vi "CANOpen_Scan Device List.vi"(10 "Baud Rate":T1 items=["1 Mbit/s"=0, "800 kbit/s"=1, "500 kbit/s"=2, "250 kbit/s"=3, "125 kbit/s"=4, "50 kbit/s"=6, "20 kbit/s"=7, "10 kbit/s"=8], 11 "CANOpen Interface Name":T2 items=["CANopen01", "CANopen02", "CANopen03", "CANopen04", "CANopen05", "CANopen06", "CANopen07", "CANopen08", "CANopen09", "CANopen10", "CANopen11", "CANopen12", "CANopen13", "CANopen14", "CANopen15", "CANopen16", "CANopen17", "CANopen18", "CANopen19", "CANopen20", "CANopen21", "CANopen22", "CANopen23", "CANopen24", "CANopen25", "CANopen26", "CANopen27", "CANopen28", "CANopen29", "CANopen30", "CANopen31", "CANopen32"]) -> ()   [LabVIEW 2013, in "CANOpen Addon Custom Device.lvlib"]
uses:
  CANOpen Addon Custom Device.lvlib
  Shared Code/CANOpen Interface Name.ctl
  <vilib>/CANopenLib/CANOPEN.llb/CANopen BaudRate.ctl
  <vilib>/CANopenLib/CANOPEN.llb/CANopen Interface Close.vi
  <vilib>/CANopenLib/CANOPEN.llb/CANopen Interface Create.vi
  <vilib>/CANopenLib/CANOPEN.llb/CANopen SDO Create.vi
  <vilib>/CANopenLib/CANOPEN.llb/CANopen SDO Read [U32].vi
  <vilib>/CANopenLib/CANOPEN.llb/CANopen SDO Close.vi
  <vilib>/CANopenLib/CANOPEN.llb/CANopen SDO Read [STR].vi
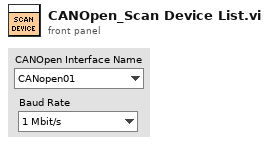
[diagram p1: front panel]
types:
  T1 = typedef "CANopen BaudRate.ctl" = u32
  T2 = typedef "CANOpen Addon Custom Device.lvlib/CANOpen Interface Name.ctl" = u32
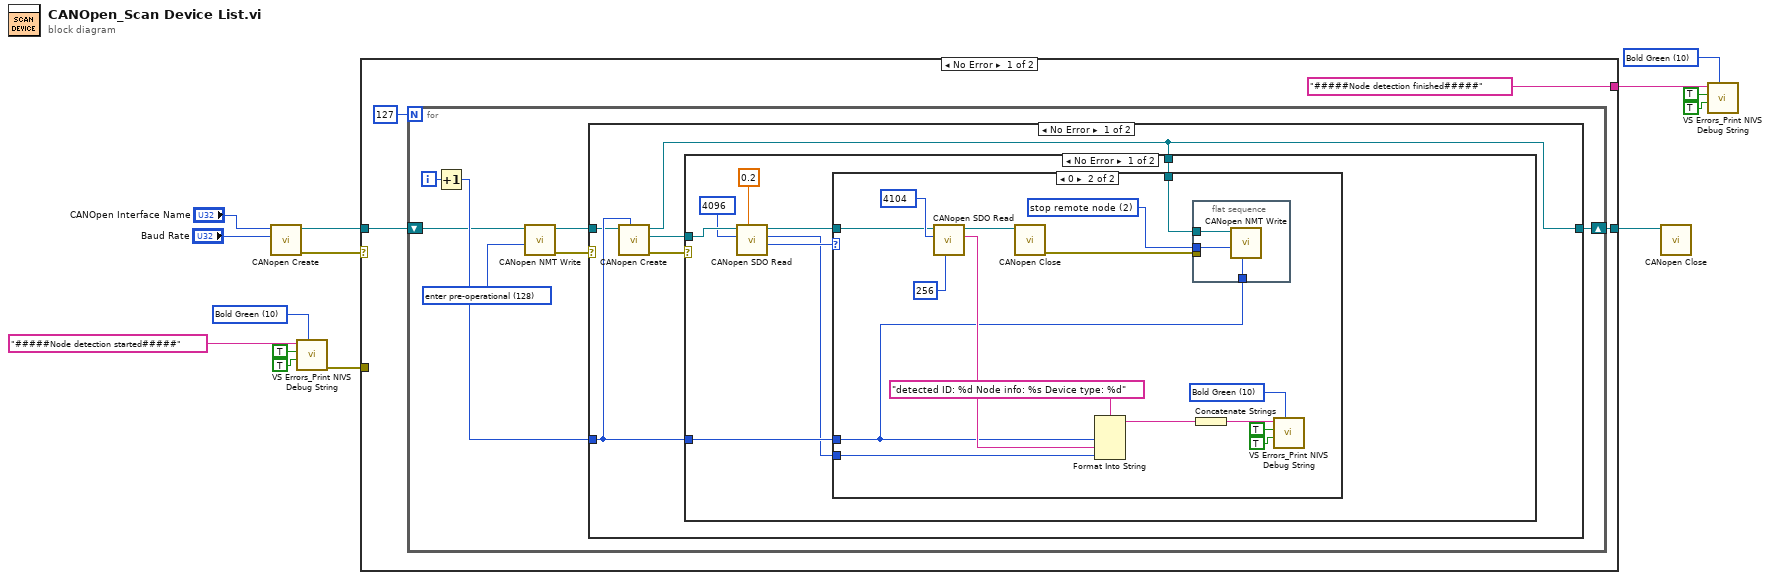
[diagram p0: block diagram]
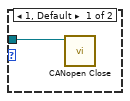
[diagram p2: hidden frame]
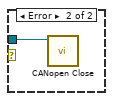
[diagram p3: hidden frame]
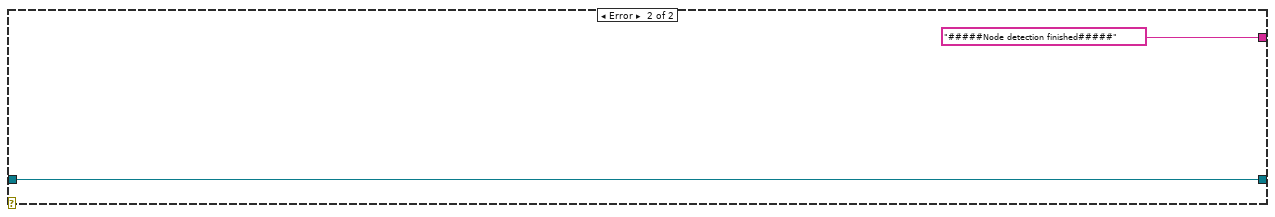
[diagram p5: hidden frame]
diagram:
  w4 = u16 10 items=["Plain White"=7, "Bold White"=15, "Bold Blue"=9, "Bold Green"=10, "Bold Red"=12] ("Color (Plain White)")
  w6 = u16 10 items=["Plain White"=7, "Bold White"=15, "Bold Blue"=9, "Bold Green"=10, "Bold Red"=12] ("Color (Plain White)")
  n1 = call-poly <vilib>:"CANopen Create.vi"("baud rate"="Baud Rate", "interface name"="CANOpen Interface Name") -> ("error out"=w10:errorcluster, "interface object out"=w12:refnum<k20>)  [unwired: 8 in]
  n2 = call "VS Errors_Print NIVS Debug String.vi"("Color (Plain White)"=w6, "Add to NIVS Log FIle? (T)"=TRUE, "Append EOL? (T)"=TRUE, "Debug String"="#####Node detection started#####") -> ("error out"=w7:errorcluster)  [unwired: 6 in]
  n3 = case shown="No Error" w10 {
    tunnel: w12 -> [w18 w62]
    tunnel: [w16 w62] -> w11
    tunnel: w7 -> [_ _]
    tunnel: ["#####Node detection finished#####" ("Debug String") "#####Node detection finished#####" ("Debug String")] -> w1
    frame No Error {
      n4 = for {
        N: 127 -> [_]
        shift-right: [w19] -> w16
        shift-left: w18 -> [w21]
        i -> [w25]
        w23 = u16 128 items=["start remote node"=1, "stop remote node"=2, "enter pre-operational"=128, "reset node"=129, "reset communication"=130] ("command")
        n5 = Increment(x=w25) -> (x+1=w24:i32)
        n6 = call <vilib>:"CANopen NMT Write.vi"("command"=w23, "interface object in"=w21) -> ("error out"=w20:errorcluster, "interface object out"=w22:refnum<k20>)  [unwired: 8 in]
        n7 = case shown="No Error" w20 {
          tunnel: w24 -> [w30 _]
          tunnel: w22 -> [w29 w60]
          tunnel: [w26 w60] -> w19
          frame No Error {
            n8 = call-poly <vilib>:"CANopen Create.vi"("node-ID"=w30, "interface object in"=w29) -> ("error out"=w27:errorcluster, "SDO object out"=w28:refnum<k20>, "interface object out"=w26:refnum<k20>)  [unwired: 7 in]
            n9 = case shown="No Error" w27 {
              tunnel: w30 -> [w38 _]
              tunnel: w28 -> [w37 w59]
              tunnel: w26 -> [w33 _]
              frame No Error {
                n10 = call-poly <vilib>:"CANopen SDO Read.vi"("timeout (1s)"=0.2, "object index"=u16 4096 ("Object Index"), "SDO object in"=w37) -> ("completion code"=w32:u32, "U32 data"=w31:u32, "SDO object out"=w34:refnum<k20>)  [unwired: 5 in, 1 out]
                n11 = case shown="0" w32 {
                  tunnel: w38 -> [_ w41]
                  tunnel: w34 -> [w39 w46]
                  tunnel: w33 -> [_ w43]
                  tunnel: w31 -> [_ w40]
                  frame 1, Default {
                    n12 = call-poly <vilib>:"CANopen Close.vi"("SDO object in"=w39) -> ()  [unwired: 10 in, 1 out]
                  }
                  frame 0 {
                    w42 = u16 2 items=["start remote node"=1, "stop remote node"=2, "enter pre-operational"=128, "reset node"=129, "reset communication"=130] ("command")
                    w53 = u16 10 items=["Plain White"=7, "Bold White"=15, "Bold Blue"=9, "Bold Green"=10, "Bold Red"=12] ("Color (Plain White)")
                    n13 = call-poly <vilib>:"CANopen SDO Read.vi"("data size"=u32 256, "object index"=u16 4104 ("Object Index"), "SDO object in"=w46) -> ("string data"=w45:string, "SDO object out"=w47:refnum<k20>)  [unwired: 5 in, 2 out]
                    n14 = call-poly <vilib>:"CANopen Close.vi"("SDO object in"=w47) -> ("error out"=w44:errorcluster)  [unwired: 10 in]
                    n15 = Format Into String(format string="detected ID: %d Node info: %s Device type: %d", w41, w45, w40) -> (resulting string=w54:string)  [unwired: 2 in, 1 out]
                    n16 = flat-sequence {
                      tunnel: w44 -> [_]
                      tunnel: w43 -> [w58]
                      tunnel: w42 -> [w57]
                      tunnel: w41 -> [w56]
                      frame #0 {
                        n17 = call <vilib>:"CANopen NMT Write.vi"("node-ID (0)"=w56, "command"=w57, "interface object in"=w58) -> ()  [unwired: 7 in, 2 out]
                      }
                    }
                    n18 = Concatenate Strings(w54) -> (w50:string)
                    n19 = call "VS Errors_Print NIVS Debug String.vi"("Color (Plain White)"=w53, "Add to NIVS Log FIle? (T)"=TRUE, "Append EOL? (T)"=TRUE, "Debug String"=w50) -> ()  [unwired: 6 in, 1 out]
                  }
                }
              }
              frame Error {
                n20 = call-poly <vilib>:"CANopen Close.vi"("SDO object in"=w59) -> ()  [unwired: 10 in, 1 out]
              }
            }
          }
          frame Error {
          }
        }
      }
    }
    frame Error {
    }
  }
  n21 = call-poly <vilib>:"CANopen Close.vi"("interface object in"=w11) -> ()  [unwired: 10 in, 1 out]
  n22 = call "VS Errors_Print NIVS Debug String.vi"("Color (Plain White)"=w4, "Add to NIVS Log FIle? (T)"=TRUE, "Append EOL? (T)"=TRUE, "Debug String"=w1) -> ()  [unwired: 6 in, 1 out]
